vi "Parse Status Response.vi"(8 "error in":errorcluster, 11 "EF20 in":refnum<class "EF20.lvclass">) -> (0 "error out":errorcluster, 3 "EF20 out":refnum<class "EF20.lvclass">)   [LabVIEW 2018, in "EF20.lvlib" / "EF20.lvclass"]
uses:
  EF20.lvclass
  EF20.lvclass/EF20.ctl
  PPLs/Oven/Oven.lvlibp/Oven.lvclass
  C:/Projects/LabVIEW/PPLs/Oven/Oven.lvlibp/Oven.lvclass
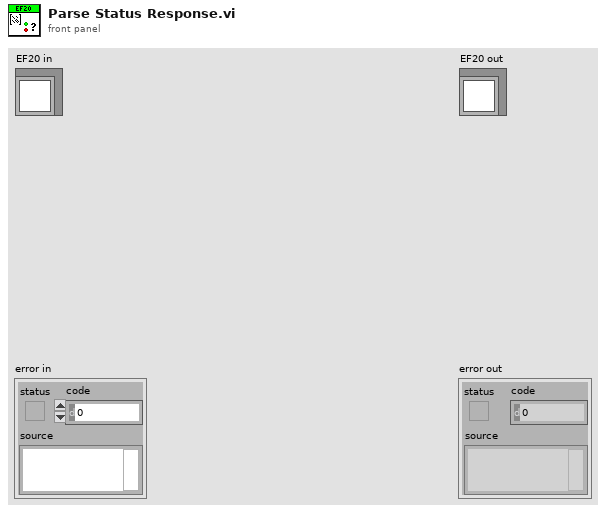
[diagram p1: front panel]
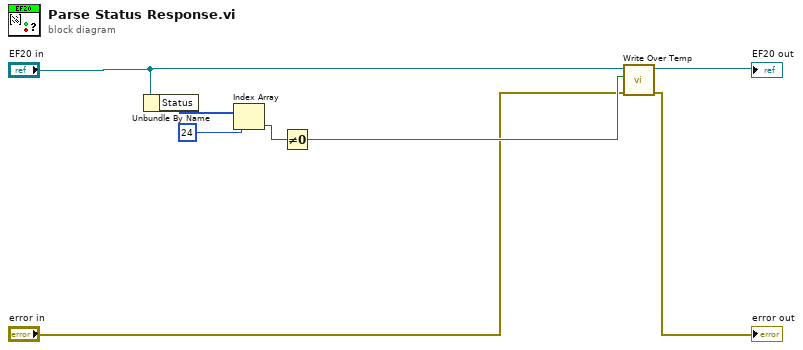
[diagram p0: block diagram]
diagram:
  n1 = Unbundle By Name("EF20 in") -> ("Status"=w5:u8[])
  n2 = Index Array(array=w5, index=24) -> (element=w7:u8)
  n3 = Not Equal To 0?(x=w7) -> (x != 0?=w8:bool)
  n4 = call "Write Over Temp.vi"("error in (no error)"="error in", "Over Temp"=w8, "Oven in"="EF20 in") -> ("error out"=→"error out":errorcluster, "Oven out"=→"EF20 out":refnum<class "EF20.lvclass">)  [unwired: 7 in]
